vi "Parameter to encoder value.vi"(8 "error in (no error)":errorcluster, 9 "parameter":string, 11 "Motor in":refnum<class "Motor.lvclass">) -> (0 "error out":errorcluster, 1 "encoder value":dbl, 2 "valid":bool, 3 "Motor out":refnum<class "Motor.lvclass">)   [LabVIEW 2018, in "Motor.lvclass"]
uses:
  Motor.lvclass
  Motor.lvclass/Motor.ctl
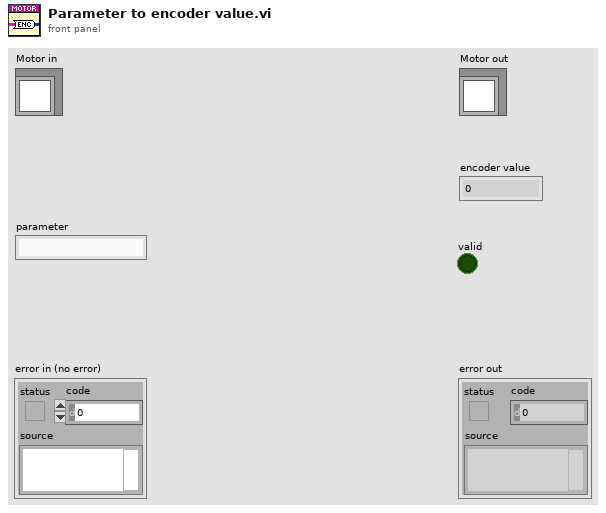
[diagram p1: front panel]
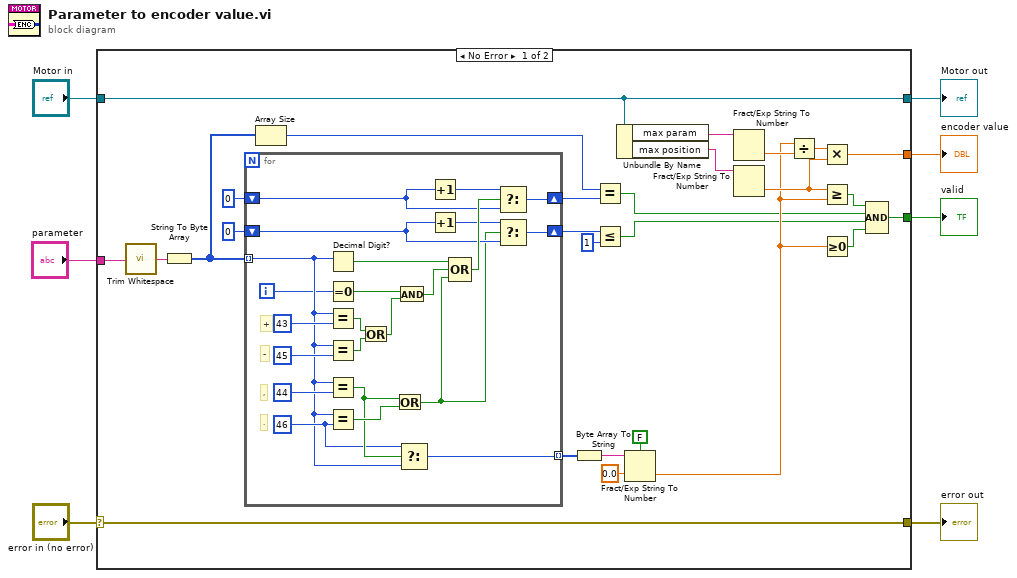
[diagram p0: block diagram]
diagram:
  n1 = case shown="No Error" "error in (no error)" {
    selector: "error in (no error)" -> [w34 w58]
    tunnel: [w34 w58] -> w6
    tunnel: [w33 w59] -> w4
    tunnel: "Motor in" -> [w33 w59]
    tunnel: [w28 _] -> w3
    tunnel: [w15 _] -> w2
    tunnel: "parameter" -> [w14 _]
    frame No Error {
      n2 = call <vilib>:"Trim Whitespace.vi"("string"=w14) -> ("trimmed string"=w26:string)  [unwired: 1 in]
      n3 = String To Byte Array(string=w26) -> (unsigned byte array=w24:u8[])
      n4 = for {
        tunnel: w24 -> [w42] mode=indexing
        shift-right: [w54] -> w20
        shift-left: 0 -> [w52]
        tunnel: [w49] -> w23 mode=indexing
        shift-right: [w47] -> w21
        shift-left: 0 -> [w46]
        i -> [w41]
        w50 = u8 46 ("y")
        # "-"
        # "+"
        # "."
        # ","
        n5 = Decimal Digit?(1:w42) -> (0:w36:bool)
        n6 = Equal To 0?(x=w41) -> (x = 0?=w38:bool)
        n7 = Equal?(x=w42, y=u8 43) -> (x = y?=w39:bool)
        n8 = Equal?(x=w42, y=u8 45) -> (x = y?=w40:bool)
        n9 = Equal?(x=w42, y=u8 44) -> (x = y?=w51:bool)
        n10 = Equal?(x=w42, y=w50) -> (x = y?=w57:bool)
        n11 = Or(x=w39, y=w40) -> (x .or. y?=w37:bool)
        n12 = Or(x=w51, y=w57) -> (x .or. y?=w45:bool)
        n13 = And(x=w38, y=w37) -> (x .and. y?=w35:bool)
        n14 = Select(t=w50, s=w51, f=w42) -> (s? t:f=w49:u8)
        n15 = Increment(x=w52) -> (x+1=w53:i32)
        n16 = Increment(x=w46) -> (x+1=w48:i32)
        n17 = Compound Arithmetic op=OR(w36, w35, w45) -> (w55:bool)
        n18 = Select(t=w53, s=w55, f=w52) -> (s? t:f=w54:i32)
        n19 = Select(t=w48, s=w45, f=w46) -> (s? t:f=w47:i32)
      }
      n20 = Array Size(array=w24) -> (size(s)=w19:i32)
      n21 = Byte Array To String(unsigned byte array=w23) -> (string=w16:string)
      n22 = Equal?(x=w19, y=w20) -> (x = y?=w8:bool)
      n23 = Less Or Equal?(x=w21, y=1) -> (x <= y?=w9:bool)
      n24 = Unbundle By Name(w33) -> ("max param"=w31:string, "max position"=w30:string)
      n25 = Fract/Exp String To Number(use system decimal point (T)=FALSE, string=w16, default (0 dbl)=0.0) -> (number=w11:dbl)  [unwired: 1 in, 1 out]
      n26 = Fract/Exp String To Number(string=w31) -> (number=w29:dbl)  [unwired: 3 in, 1 out]
      n27 = Fract/Exp String To Number(string=w30) -> (number=w12:dbl)  [unwired: 3 in, 1 out]
      n28 = Divide(x=w11, y=w29) -> (x/y=w32:dbl)
      n29 = Multiply(x=w32, y=w12) -> (x*y=w28:dbl)
      n30 = Greater Or Equal?(x=w12, y=w11) -> (x >= y?=w10:bool)
      n31 = Greater Or Equal To 0?(x=w11) -> (x >= 0?=w13:bool)
      n32 = Compound Arithmetic op=AND(w10, w8, w9, w13) -> (w15:bool)
    }
    frame Error {
    }
  }
  "error out" <- w6
  "Motor out" <- w4
  "valid" <- w2
  "encoder value" <- w3
